vi "ellipse parameters from points svd.vi"(10 "y":dbl[](array[numeric]) format="%0.2f", 11 "X":dbl[](array[numeric]) format="%0.2f") -> (3 "ellipse parameters":T1)   [LabVIEW 2017]
uses:
  <vilib>/Analysis/7linalg.llb/SVD Option.ctl
  <vilib>/Analysis/baseanly.llb/Mean (DBL).vi
  <vilib>/Analysis/7linalg.llb/Real SVD Decomposition.vi
  <vilib>/Analysis/NI_AALBase.lvlib
  <vilib>/Analysis/NI_AALPro.lvlib
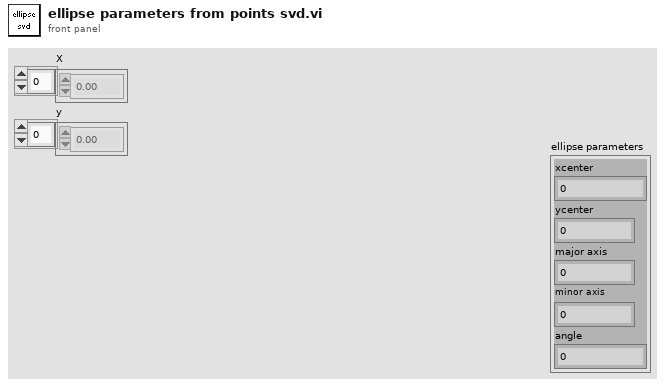
[diagram p1: front panel]
types:
  T1 = cluster{"xcenter":dbl, "ycenter":dbl, "major axis":dbl, "minor axis":dbl, "angle":dbl}
  T2 = typedef "NI_AALPro.lvlib/SVD Option.ctl" = u16
  T3 = typedef "NI_Matrix.lvlib/RealMatrix.ctl" = dbl[][]
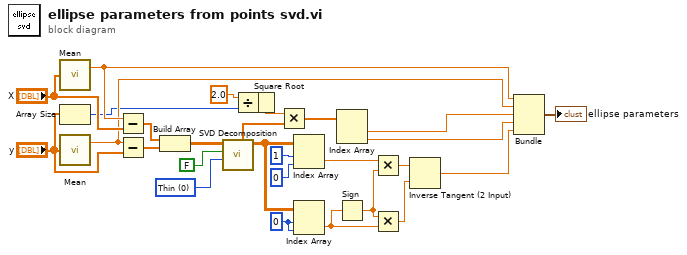
[diagram p0: block diagram]
diagram:
  w22 = 0 ("index (row)")
  w23 = T2 0 items=["Thin", "Full"] ("SVD option")
  n1 = call-poly <vilib>:"Mean.vi"("X"="X") -> ("mean"=w12:dbl)  [unwired: 1 out]
  n2 = Array Size(array="y") -> (size(s)=w4:i32)
  n3 = call-poly <vilib>:"Mean.vi"("X"="y") -> ("mean"=w11:dbl)  [unwired: 1 out]
  n4 = Subtract(x=w12, y="X") -> (x-y=w27:dbl[])
  n5 = Subtract(x=w11, y="y") -> (x-y=w26:dbl[])
  n6 = Build Array(w27, w26) -> (w25:dbl[][])
  n7 = call-poly <vilib>:"SVD Decomposition.vi"("SVD option"=w23, "singular values only?"=FALSE, "A"=w25) -> ("Matrix U"=w21:T3, "Vector S"=w13:dbl[])  [unwired: 4 in, 3 out]
  n8 = Divide(x=2.0, y=w4) -> (x/y=w3:dbl)
  n9 = Square Root(x=w3) -> (sqrt(x)=w1:dbl)
  n10 = Multiply(x=w1, y=w13) -> (x*y=w2:dbl[])
  n11 = Index Array(array=w21, index (row)=1, index (col)=0) -> (element=w18:dbl)
  n12 = Index Array(array=w21, index (row)=w22, index (col)=w22) -> (element=w17:dbl)
  n13 = Index Array(array=w2) -> (element #1=w10:dbl, element #2=w9:dbl)  [unwired: 2 in]
  n14 = Sign(1:w17) -> (0:w14:dbl)
  n15 = Multiply(x=w18, y=w14) -> (x*y=w15:dbl)
  n16 = Multiply(x=w14, y=w17) -> (x*y=w16:dbl)
  n17 = Inverse Tangent (2 Input)(1:w16, 2:w15) -> (0:w8:dbl)
  n18 = Bundle("mean"=w12, "mean"=w11, w10, w9, w8) -> (→"ellipse parameters":cluster{"mean":dbl, "mean":dbl, dbl, dbl, dbl})  [unwired: 1 in]
